vi "copyFileToRunDir.vi"(8 "error in (no error)":errorcluster, 10 "Path":path, 11 "FileNeologist in":refnum<class "FileNeologist.lvclass">) -> (0 "error out":errorcluster, 3 "FileNeologist out":refnum<class "FileNeologist.lvclass">)   [LabVIEW 2011, in "Tools.lvlib" / "Filing.lvlib" / "FileNeologist.lvclass"]
doc: "Copy this file to the run directory."
uses:
  FileNeologist.lvclass
  FileNeologist.lvclass/FileNeologist.ctl
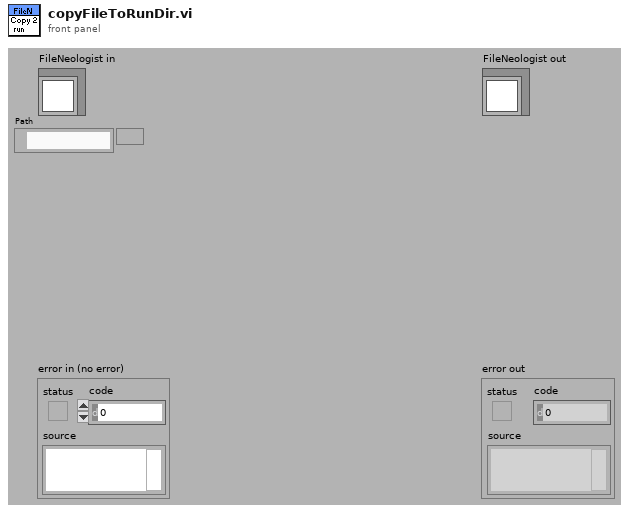
[diagram p1: front panel]
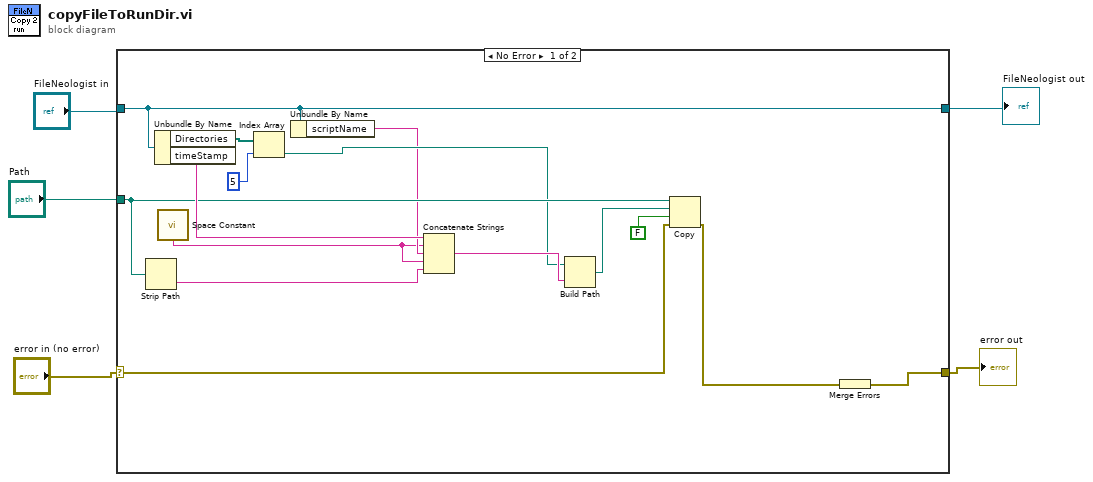
[diagram p0: block diagram]
diagram:
  n1 = case shown="No Error" "error in (no error)" {
    selector: "error in (no error)" -> [w10 w22]
    tunnel: [w17 w22] -> w2
    tunnel: [w9 w21] -> w5
    tunnel: "FileNeologist in" -> [w9 w21]
    tunnel: "Path" -> [w13 _]
    frame No Error {
      n2 = Strip Path(path=w13) -> (name=w6:string)  [unwired: 1 out]
      n3 = Unbundle By Name(w9) -> ("Directories"=w14:path[], "timeStamp"=w18:string)
      n4 = call <vilib>:"Space Constant.vi"() -> ("String"=w7:string)
      n5 = Index Array(array=w14, index=5) -> (element=w11:path)
      n6 = Unbundle By Name(w9) -> ("scriptName"=w8:string)
      n7 = Concatenate Strings(w18, w7, w8, w7, w6) -> (w15:string)
      n8 = Build Path(base path=w11, name or relative path=w15) -> (appended path=w19:path)
      n9 = Copy(8:w10, 9:FALSE, 10:w19, 11:w13) -> (0:w16:errorcluster)  [unwired: 1 in, 2 out]
      n10 = Merge Errors(w16) -> (w17:errorcluster)
    }
    frame Error {
    }
  }
  "error out" <- w2
  "FileNeologist out" <- w5
